vi "time2mm001.vi"(1 "reverse?":bool, 2 "Offset (mm)":dbl, 3 "time":dbl) -> (0 "position (mm)":dbl)   [LabVIEW 2020]
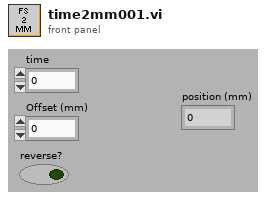
[diagram p1: front panel]
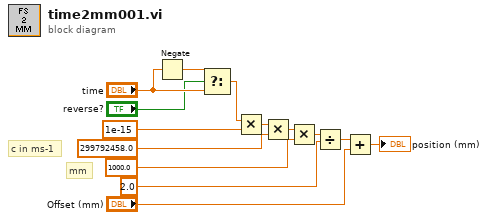
[diagram p0: block diagram]
diagram:
  # "mm"
  # "c in ms-1"
  n1 = Negate(x="time") -> (-x=w3:dbl)
  n2 = Select(t=w3, s="reverse?", f="time") -> (s? t:f=w4:dbl)
  n3 = Multiply(x=w4, y=1e-15) -> (x*y=w5:dbl)
  n4 = Multiply(x=w5, y=299792458.0) -> (x*y=w7:dbl)
  n5 = Multiply(x=w7, y=1000.0) -> (x*y=w9:dbl)
  n6 = Divide(x=w9, y=2.0) -> (x/y=w12:dbl)
  n7 = Add(x=w12, y="Offset (mm)") -> (x+y=→"position (mm)":dbl)
